vi "FTW-SEQ-Current.vi"(1 "FTW Job Sequencer":refnum<class "FTW-JobSequencer.lvclass">) -> (0 "Current Job":string)   [LabVIEW 2012, in "FTW-Actor.lvlib" / "FTW-JobSequencer.lvclass"]
uses:
  FTW-JobSequencer.lvclass
  FTW-JobSequencer.lvclass/FTW-JobSequencer.ctl
panel:
  # "Inputs"
  # "Outputs"
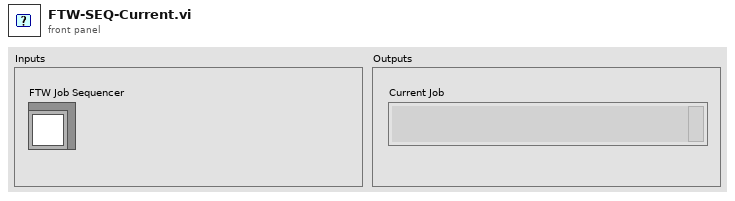
[diagram p1: front panel]
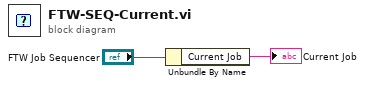
[diagram p0: block diagram]
diagram:
  n1 = Unbundle By Name("FTW Job Sequencer") -> ("Current Job"=→"Current Job":string)
